vi "Save File Common Headers.vi"(8 "Error In":errorcluster, 11 "Appliance Details":T1 {"Dryer"."Dryer Initial IMC Data"."Maximum Weight (lbf)" format="%03_6g"; "Dryer"."Dryer Initial IMC Data"."Average Weight (lbf)" format="%03_6g"; "Dryer"."Dryer Initial IMC Data"."Minimum Weight (lbf)" format="%03_6g"; "Dryer"."Dryer Initial IMC Data"."CEF (lbf/kWh)" format="%03_6g"; "Dryer"."Dryer Initial IMC Data"."Actual Final RMC (%)" format="%03_6g"; "Dryer"."Dryer Initial IMC Data"."Tolerance(%)" format="%0#_6g"; "Dryer"."Dryer Initial IMC Data"."Bone Dry Wt(lbs)" format="%03_6g"; "Dryer"."Dryer Initial IMC Data"."RMC (Desired %)" format="%0#_6g"; "Dryer"."Dryer Initial IMC Data"."Actual Initial RMC (%)" format="%03_6g"; "Dryer"."Dryer Initial IMC Data"."Measured IMC (lbs)" format="%0#_6g"}) -> (0 "Error Out":errorcluster, 3 "array":string[][](array[string]))   [LabVIEW 2018, in "File Setup.lvlib"]
uses:
  File Setup.lvlib
  File Setup (Public)/Type Definition/Save File DISH Dishwasher Details.ctl
  <vilib>/Platform/fileVersionInfo.llb/FileVersionInformation.ctl
  Washer DOE/Type Definitions/DOE Appliance Common.ctl
  Custom Pallet Controls/Custom Pallet String.ctl
  File Setup (Public)/Type Definition/DPT IMC Data.ctl
  Washer DOE/Type Definitions/DOE Dryer Standard.ctl
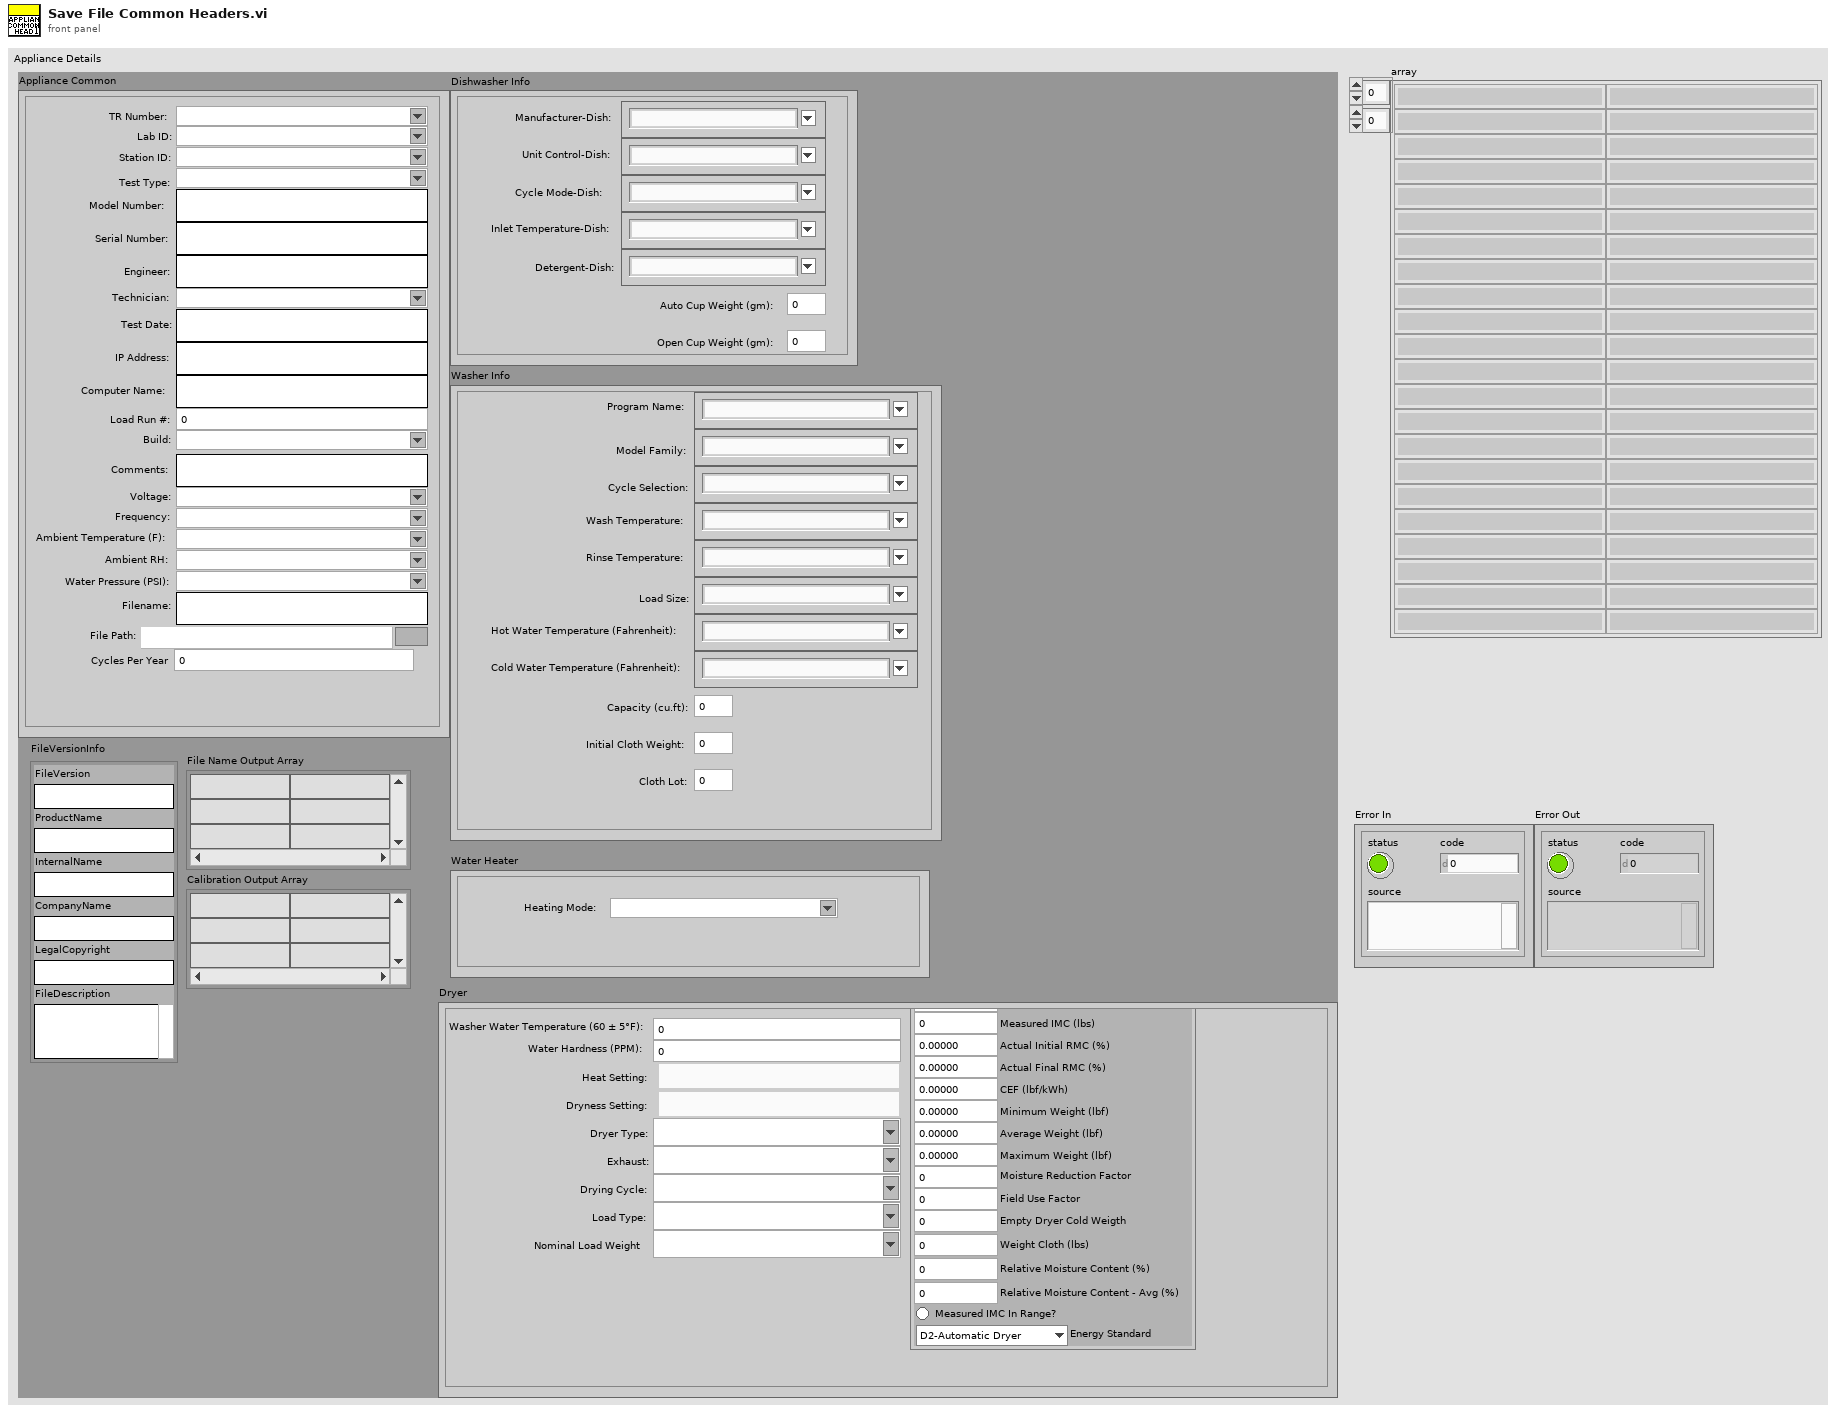
[diagram p1: front panel]
types:
  T1 = typedef "File Setup.lvlib/Save File DISH Dishwasher Details.ctl" = cluster{"FileVersionInfo":T2, "Dishwasher Info":cluster{"Open Cup Weight (gm):":dbl, "Auto Cup Weight (gm):":dbl, "Detergent-Dish:":string, "Inlet Temperature-Dish:":string, "Cycle Mode-Dish:":string, "Unit Control-Dish:":string, "Manufacturer-Dish:":string}, "Washer Info":cluster{"Hot Water Temperature (Fahrenheit):":string, "Cold Water Temperature (Fahrenheit):":string, "Capacity (cu.ft):":dbl, "Initial Cloth Weight:":dbl, "Cloth Lot:":i32, "Model Family:":string, "Program Name:":string, "Cycle Selection:":string, "Wash Temperature:":string, "Rinse Temperature:":string, "Load Size:":string}, "File Name Output Array":string[][], "Calibration Output Array":string[][], "Appliance Common":T3, "Water Heater":cluster{"Heating Mode:":string}, "Dryer":cluster{"Heat Setting:":T4, "Washer Water Temperature (60 ± 5°F):":u16, "Water Hardness (PPM):":u16, "Dryness Setting:":T4, "Dryer Type:":string, "Exhaust:":string, "Drying Cycle:":string, "Load Type:":string, "Nominal Load Weight":string, "Dryer Initial IMC Data":T5}}
  T2 = typedef "FileVersionInformation.ctl" = cluster{"FileVersion":string, "ProductName":string, "InternalName":string, "CompanyName":string, "LegalCopyright":string, "FileDescription":string}
  T3 = typedef "DOE Appliance Common.ctl" = cluster{"Engineer:":string, "Model Number:":string, "Serial Number:":string, "Comments:":string, "Station ID:":string, "Technician:":string, "TR Number:":string, "Lab ID:":string, "Voltage:":string, "Water Pressure (PSI):":string, "Test Date:":string, "Computer Name:":string, "IP Address:":string, "Ambient RH:":string, "Frequency:":string, "Build:":string, "Filename:":string, "Test Type:":string, "Load Run #:":i32, "Ambient Temperature (F):":string, "File Path:":path, "Cycles Per Year":u32}
  T4 = typedef "Custom Pallet String.ctl" = string
  T5 = typedef "DPT IMC Data.ctl" = cluster{"Measured IMC (lbs)":dbl, "Actual Initial RMC (%)":dbl, "RMC (Desired %)":dbl, "Bone Dry Wt(lbs)":dbl, "Tolerance(%)":dbl, "Actual Final RMC (%)":dbl, "CEF (lbf/kWh)":dbl, "Minimum Weight (lbf)":dbl, "Average Weight (lbf)":dbl, "Maximum Weight (lbf)":dbl, "Measured IMC In Range?":bool, "Moisture Reduction Factor":dbl, "Field Use Factor":dbl, "Empty Dryer Cold Weigth":dbl, "Energy Standard":T6, "Weight Cloth (lbs)":dbl, "Relative Moisture Content (%)":dbl, "Relative Moisture Content - Avg (%)":dbl}
  T6 = typedef "DOE Dryer Standard.ctl" = enum16{"D2-Automatic Dryer", "D2-Timer Dryer", "D1-Automatic Dryer", "D1-Timer Dryer", "Other"}
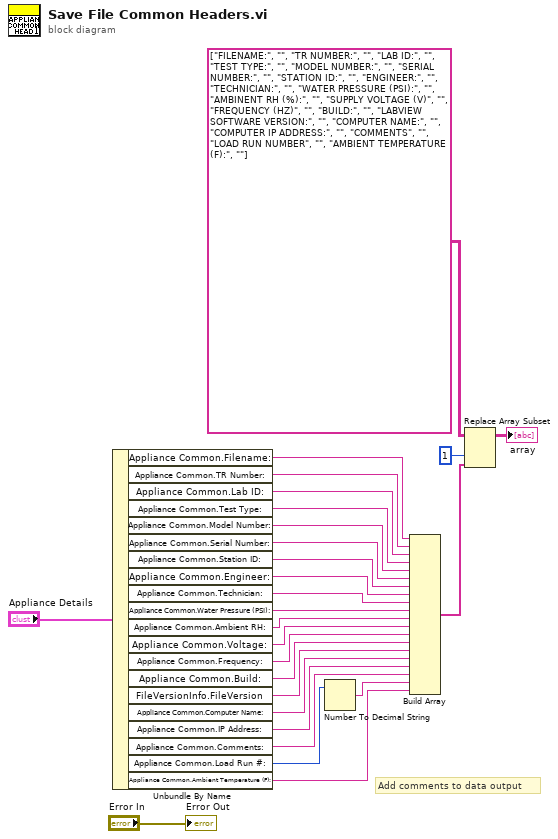
[diagram p0: block diagram]
diagram:
  # "Add comments to data output"
  n1 = Unbundle By Name("Appliance Details") -> ("Appliance Common.Filename:"=w4:string, "Appliance Common.TR Number:"=w5:string, "Appliance Common.Lab ID:"=w6:string, "Appliance Common.Test Type:"=w24:string, "Appliance Common.Model Number:"=w7:string, "Appliance Common.Serial Number:"=w8:string, "Appliance Common.Station ID:"=w9:string, "Appliance Common.Engineer:"=w10:string, "Appliance Common.Technician:"=w11:string, "Appliance Common.Water Pressure (PSI):"=w12:string, "Appliance Common.Ambient RH:"=w13:string, "Appliance Common.Voltage:"=w14:string, "Appliance Common.Frequency:"=w15:string, "Appliance Common.Build:"=w16:string, "FileVersionInfo.FileVersion"=w17:string, "Appliance Common.Computer Name:"=w18:string, "Appliance Common.IP Address:"=w19:string, "Appliance Common.Comments:"=w20:string, "Appliance Common.Load Run #:"=w25:i32, "Appliance Common.Ambient Temperature (F):"=w27:string)
  n2 = Number To Decimal String(number=w25) -> (decimal integer string=w26:string)  [unwired: 1 in]
  n3 = Build Array(w4, w5, w6, w24, w7, w8, w9, w10, w11, w12, w13, w14, w15, w16, w17, w18, w19, w20, w26, w27) -> (w22:string[])
  n4 = Replace Array Subset(array=string[][] [["FILENAME:", ""], ["TR NUMBER:", ""], ["LAB ID:", ""], ["TEST TYPE:", ""], ["MODEL NUMBER:", ""], ["SERIAL NUMBER:", ""], ["STATION ID:", ""], ["ENGINEER:", ""], ["TECHNICIAN:", ""], ["WATER PRESSURE (PSI):", ""], ["AMBINENT RH (%):", ""], ["SUPPLY VOLTAGE (V)", ""], ["FREQUENCY (HZ)", ""], ["BUILD:", ""], ["LABVIEW SOFTWARE VERSION:", ""], ["COMPUTER NAME:", ""], ["COMPUTER IP ADDRESS:", ""], ["COMMENTS", ""], ["LOAD RUN NUMBER", ""], ["AMBIENT TEMPERATURE (F):", ""]], new element=w22, index (col)=1 ("disabled index (col)")) -> (→"array":string[][])  [unwired: 1 in]
  "Error Out" <- "Error In"
